vi "Import Resources.vi"(7 "Ignore New? (F)":bool, 9 "Resources []":T1[](array[typedef]), 10 "Languages []":T2[](array[typedef]), 11 "LangFile.lvclass in":refnum<class "Resource Data.lvclass">) -> (3 "LangFile.lvclass out":refnum<class "Resource Data.lvclass">)   [LabVIEW 2013, in "SET Project Data.lvlib" / "Resource Data.lvclass"]
uses:
  Resource Data.lvclass
  Types/ProjFile_Language Entry.ctl
  Types/ProjFile_Resource Entry.ctl
  Resource Data.lvclass/Resource Data.ctl
  SET Project Data.lvlib
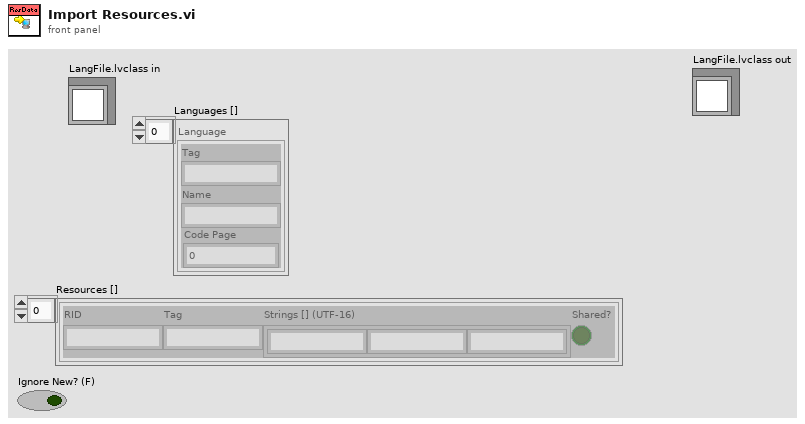
[diagram p1: front panel]
types:
  T1 = typedef "SET Project Data.lvlib/ProjFile_Resource Entry.ctl" = cluster{"RID":string, "Tag":string, "Strings [] (UTF-16)":string[], "Shared?":bool}
  T2 = typedef "SET Project Data.lvlib/ProjFile_Language Entry.ctl" = cluster{"Tag":string, "Name":string, "Code Page":u16}
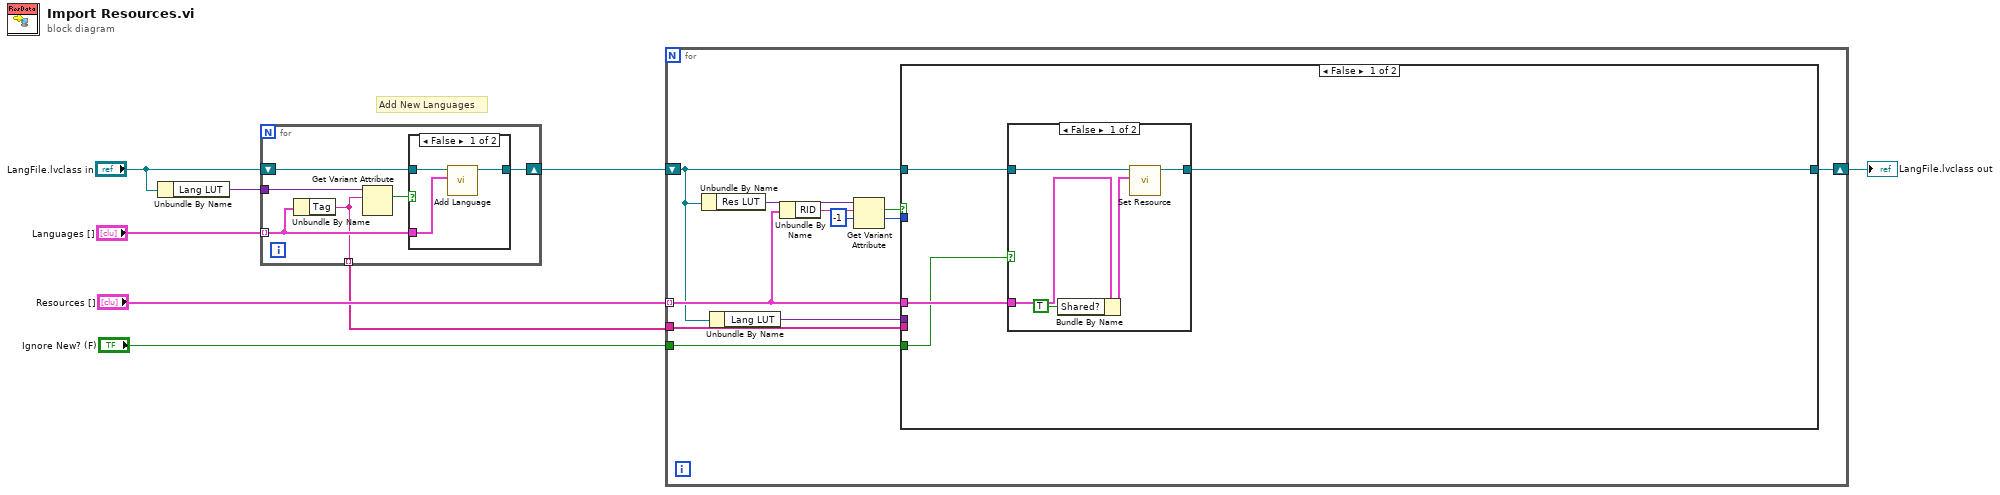
[diagram p0: block diagram]
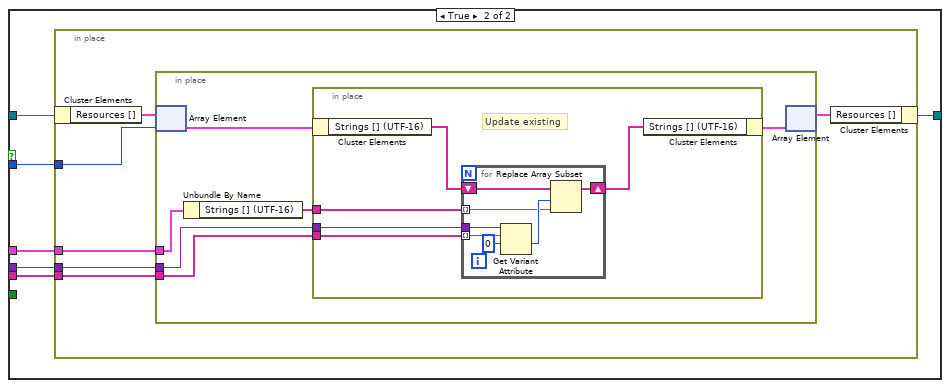
[diagram p3: hidden frame]
diagram:
  # "Add New Languages"
  n1 = Unbundle By Name("LangFile.lvclass in") -> ("Lang LUT"=w7:variant)
  n2 = for {
    tunnel: "Languages []" -> [w10] mode=indexing
    tunnel: w7 -> [w12]
    shift-right: [w13] -> w5
    shift-left: "LangFile.lvclass in" -> [w14]
    tunnel: [w9] -> w1 mode=indexing
    n3 = Unbundle By Name(w10) -> ("Tag"=w9:string)
    n4 = Get Variant Attribute(Variant=w12, name=w9) -> (found=w11:bool)  [unwired: 2 in, 3 out]
    n5 = case shown="False" w11 {
      tunnel: w14 -> [w17 w18]
      tunnel: [w16 w18] -> w13
      tunnel: w10 -> [w15 _]
      frame False {
        n6 = call "Add Language.vi"("Language"=w15, "LangFile in"=w17) -> ("LangFile out"=w16:refnum<class "Resource Data.lvclass">)  [unwired: 8 in, 1 out]
      }
      frame True {
      }
    }
  }
  n7 = for {
    shift-right: [w22] -> w8
    shift-left: w5 -> [w20]
    tunnel: w1 -> [w29]
    tunnel: "Resources []" -> [w28] mode=indexing
    tunnel: "Ignore New? (F)" -> [w21]
    n8 = Unbundle By Name(w20) -> ("Res LUT"=w27:variant)
    n9 = Unbundle By Name(w20) -> ("Lang LUT"=w19:variant)
    n10 = Unbundle By Name(w28) -> ("RID"=w26:string)
    n11 = Get Variant Attribute(Variant=w27, name=w26, default value (empty Variant)=-1) -> (found=w23:bool, value=w24:i32)  [unwired: 1 in, 2 out]
    n12 = case shown="False" w23 {
      tunnel: w24 -> [_ w42]
      tunnel: w28 -> [w33 w45]
      tunnel: w29 -> [_ w44]
      tunnel: w19 -> [_ w43]
      tunnel: w20 -> [w32 w41]
      tunnel: [w31 w40] -> w22
      tunnel: w21 -> [w30 _]
      frame False {
        n13 = case shown="False" w30 {
          tunnel: w33 -> [w36 _]
          tunnel: w32 -> [w38 w39]
          tunnel: [w37 w39] -> w31
          frame False {
            n14 = Bundle By Name(cluster=w36, "Shared?"=TRUE) -> (w35:T1)
            n15 = call "Set Resource.vi"("Resource"=w35, "LangFile in"=w38) -> ("LangFile out"=w37:refnum<class "Resource Data.lvclass">)  [unwired: 8 in, 1 out]
          }
          frame True {
            # "Ignore New?"
          }
        }
      }
      frame True {
        n16 = in-place {
          in-place-border: w45 -> [w51]
          in-place-border: w44 -> [w50]
          in-place-border: w43 -> [w49]
          in-place-border: w42 -> [w48]
          n17 = in-place-cluster #1(w41) -> ("Resources []"=w47:T1[])
          n18 = in-place {
            in-place-border: w51 -> [w57]
            in-place-border: w50 -> [w55]
            in-place-border: w49 -> [w54]
            n19 = in-place-array #2(w47, w48) -> (w53:T1)
            n20 = Unbundle By Name(w57) -> ("Strings [] (UTF-16)"=w56:string[])
            n21 = in-place {
              in-place-border: w56 -> [w62]
              in-place-border: w55 -> [w61]
              in-place-border: w54 -> [w60]
              # "Update existing"
              n22 = in-place-cluster #3(w53) -> ("Strings [] (UTF-16)"=w59:string[])
              n23 = for {
                tunnel: w62 -> [w63] mode=indexing
                tunnel: w61 -> [w68] mode=indexing
                tunnel: w60 -> [w69]
                shift-right: [w65] -> w58
                shift-left: w59 -> [w66]
                n24 = Get Variant Attribute(Variant=w69, name=w68, default value (empty Variant)=0) -> (value=w64:i32)  [unwired: 1 in, 3 out]
                n25 = Replace Array Subset(array=w66, new element=w63, index=w64) -> (w65:string[])
              }
              n26 = in-place-cluster #3("Strings [] (UTF-16)"=w58) -> (w52:T1)
            }
            n27 = in-place-array #2(w52) -> (w46:T1[])  [unwired: 1 out]
          }
          n28 = in-place-cluster #1("Resources []"=w46) -> (w40:refnum<class "Resource Data.lvclass">)
        }
      }
    }
  }
  "LangFile.lvclass out" <- w8
